vi "Perimeter.vi"(8 "error in (no error)":errorcluster, 11 "Circle in":refnum<class "Circle.lvclass">) -> (0 "error out":errorcluster, 2 "perimeter":dbl, 3 "Circle out":refnum<class "Circle.lvclass">)   [LabVIEW 2015, in "Circle.lvclass"]
uses:
  Circle.lvclass
  Circle.lvclass/Circle.ctl
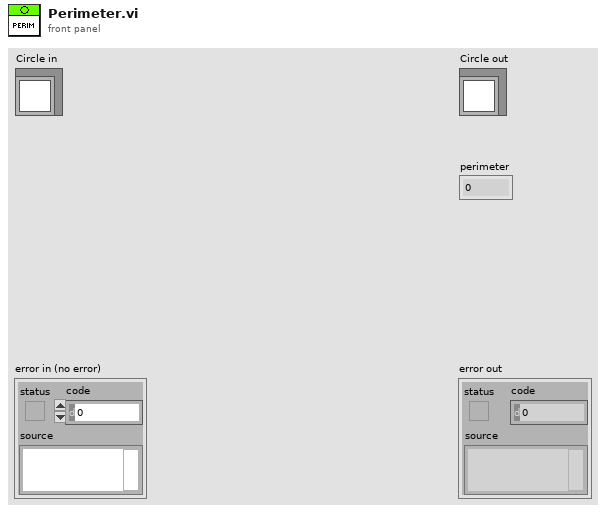
[diagram p1: front panel]
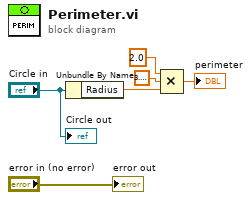
[diagram p0: block diagram]
diagram:
  n1 = Unbundle By Name("Circle in") -> ("Radius"=w5:dbl)
  n2 = Compound Arithmetic op=MULTIPLY(2.0 ("value"), 3.141592653589793, w5) -> (→"perimeter":dbl)
  "error out" <- "error in (no error)"
  "Circle out" <- "Circle in"
